vi "ClearPastColon.vi"(11 "Array in":string[](array[string])) -> (3 "Array out":string[](array[string]))   [LabVIEW 2016]
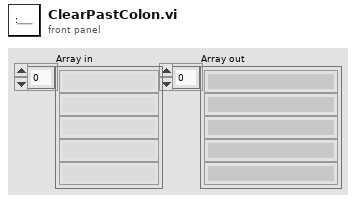
[diagram p1: front panel]
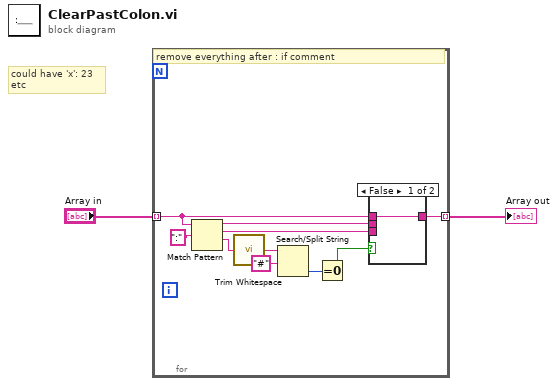
[diagram p0: block diagram]
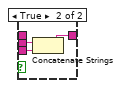
[diagram p2: hidden frame]
diagram:
  # "could have 'x': 23\netc"
  n1 = for {
    tunnel: "Array in" -> [w9] mode=indexing
    tunnel: [w10] -> w2 mode=indexing
    # "remove everything after : if comment"
    n2 = Match Pattern(string=w9, regular expression=":") -> (before substring=w8:string, match substring=w11:string, after substring=w7:string)  [unwired: 1 in, 1 out]
    n3 = call <vilib>:"Trim Whitespace.vi"("string"=w7) -> ("trimmed string"=w6:string)  [unwired: 1 in]
    n4 = Search/Split String(string=w6, search string/char (-)="#") -> (offset of match=w4:i32)  [unwired: 1 in, 2 out]
    n5 = Equal To 0?(x=w4) -> (x = 0?=w3:bool)
    n6 = case shown="False" w3 {
      tunnel: w8 -> [_ w16]
      tunnel: w11 -> [_ w15]
      tunnel: [w13 w14] -> w10
      tunnel: w9 -> [w13 _]
      frame False {
      }
      frame True {
        n7 = Concatenate Strings(w16, w15) -> (w14:string)
      }
    }
  }
  "Array out" <- w2
